vi "Arduino Write Log.vi"(7 "Msg Ref":refnum<vi>, 8 "Arduino data":string, 9 "Command":string, 10 "Message":string, 11 "log ref":refnum<file>) -> ()   [LabVIEW 2024, in "FW Arduino Control.lvclass"]
uses:
  FW Arduino Control.lvclass
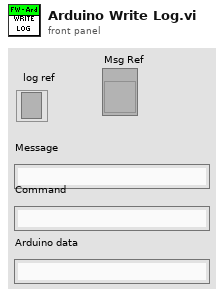
[diagram p1: front panel]
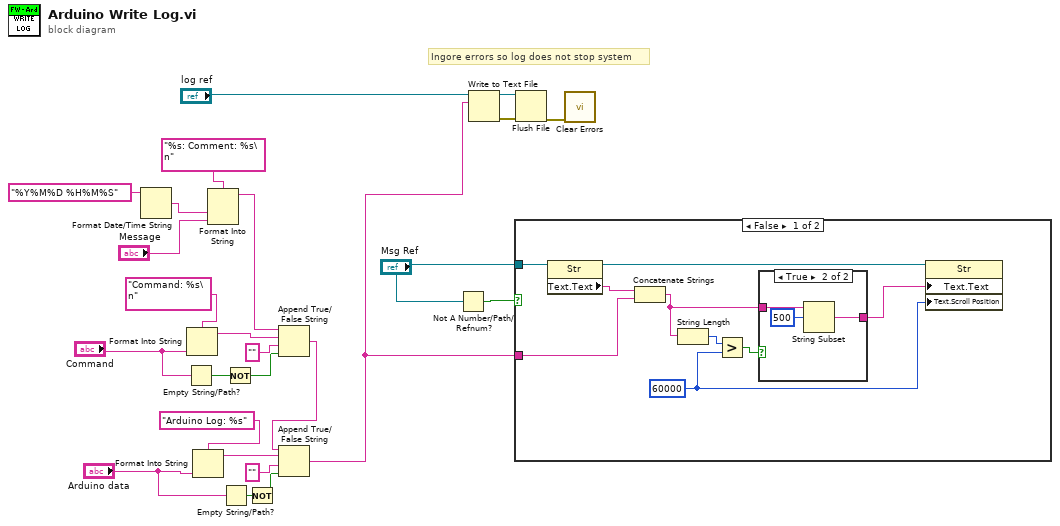
[diagram p0: block diagram]
diagram:
  # "Ingore errors so log does not stop system"
  n1 = Format Date/Time String(time format string (%c)="%Y%M%D %H%M%S") -> (date/time string=w19:string)  [unwired: 2 in]
  n2 = Empty String/Path?(string/path="Command") -> (empty?=w13:bool)
  n3 = Format Into String(format string="Command: %s\n" ("time format string (%c)"), "Command") -> (resulting string=w12:string)  [unwired: 2 in, 1 out]
  n4 = Format Into String(format string="Arduino Log: %s" ("time format string (%c)"), "Arduino data") -> (resulting string=w6:string)  [unwired: 2 in, 1 out]
  n5 = Format Into String(format string="%s: Comment: %s\n" ("time format string (%c)"), w19, "Message") -> (resulting string=w4:string)  [unwired: 2 in, 1 out]
  n6 = Empty String/Path?(string/path="Arduino data") -> (empty?=w9:bool)
  n7 = Not(x=w13) -> (.not. x?=w1:bool)
  n8 = Not(x=w9) -> (.not. x?=w2:bool)
  n9 = Append True/False String(1:w1, 2:"" ("false string"), 3:w12, 4:w4) -> (0:w5:string)
  n10 = Append True/False String(1:w2, 2:"" ("false string"), 3:w6, 4:w5) -> (0:w3:string)
  n11 = Not A Number/Path/Refnum?(number/path/refnum="Msg Ref") -> (NaN/Path/Refnum?=w17:bool)
  n12 = Write to Text File(file (use dialog)="log ref", text=w3) -> (refnum out=w23:refnum<file>, error out=w25:errorcluster)  [unwired: 2 in, 1 out]
  n13 = case shown="False" w17 {
    tunnel: "Msg Ref" -> [w34 _]
    tunnel: w3 -> [w32 _]
    frame False {
      w26 = 60000 ("y")
      n14 = property class="Str"(reference=w34) -> (reference out=w31:refnum<vi>, "Text.Text"=w33:string)  [unwired: 1 in, 1 out]
      n15 = Concatenate Strings(w33, w32) -> (w28:string)
      n16 = String Length(string=w28) -> (length=w30:i32)
      n17 = Greater?(x=w30, y=w26) -> (0:w29:bool)
      n18 = case shown="True" w29 {
        tunnel: w28 -> [w35 w38]
        tunnel: [w35 w36] -> w27
        frame False {
        }
        frame True {
          n19 = String Subset(string=w38, offset (0)=500) -> (substring=w36:string)  [unwired: 1 in]
        }
      }
      n20 = property class="Str"(reference=w31, "Text.Text"=w27, "Text.Scroll Position"=w26) -> ()  [unwired: 1 in, 2 out]
    }
    frame True {
    }
  }
  n21 = Flush File(refnum=w23, error in=w25) -> (error out=w24:errorcluster)  [unwired: 1 out]
  n22 = call <vilib>:"Clear Errors.vi"("error in (no error)"=w24) -> ()  [unwired: 5 in, 2 out]
